vi "Actor Core.vi"(8 "error in":errorcluster, 11 "Nested in":refnum<class "Coins.lvclass">) -> (0 "error out":errorcluster, 3 "Actor out":refnum<class "Actor.lvclass">)   [LabVIEW 2020, in "Coins.lvlib" / "Coins.lvclass"]
doc: "(<B>Filename</B>: Actor Framework.lvlib:Actor.lvclass:Actor Core.vi)\n\nReceives messages to the actor, reacts to them, and initiates any error handling that may shut the actor down.\n\nDescendant classes may override this VI to append parallel tasks for the actor to complete while it handles messages. Overrides use the Call Parent Method node."
uses:
  Coins.lvclass
  C:/Program Files (x86)/National Instruments/LabVIEW 2020/vi.lib/ActorFramework/Actor/Actor.lvclass
  <vilib>/ActorFramework/Actor/Actor.lvclass
  Controls/Currency Enum.ctl
  Coins.lvclass/Coins.ctl
  <vilib>/ActorFramework/Actor/Actor.lvclass/Actor.ctl
  <vilib>/ActorFramework/Message Enqueuer/Message Enqueuer.lvclass/Message Enqueuer.ctl
  Coins Messages/UpdateCoinArray Msg/UpdateCoinArray Msg.lvclass/UpdateCoinArray Msg.ctl
  Coins Messages/AddCredit Msg/AddCredit Msg.lvclass/AddCredit Msg.ctl
  <vilib>/ActorFramework/Message Enqueuer/Init from Existing Queue.vi
  <vilib>/ActorFramework/Message Enqueuer/Enqueue.vi
  <vilib>/ActorFramework/Stop Msg/Stop Msg.lvclass
  C:/Program Files (x86)/National Instruments/LabVIEW 2020/vi.lib/ActorFramework/Message/Message.lvclass
  Coins Messages/UpdateCoinArray Msg/UpdateCoinArray Msg.lvclass
  Coins Messages/AddCredit Msg/AddCredit Msg.lvclass
  Coins Messages/CancelPurchase Msg/CancelPurchase Msg.lvclass
  <vilib>/ActorFramework/Message Priority Queue/Priority Enqueue.vi
  <vilib>/ActorFramework/Message Enqueuer/Message Enqueuer.lvclass
panel:
  in  "Coins Cluster":T1
  out "Currency":T2
  in  "Cancel Button":bool
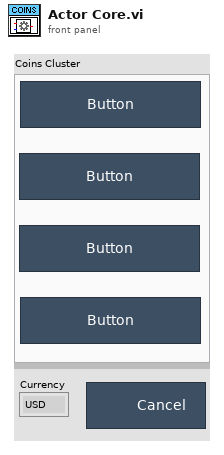
[diagram p1: front panel]
types:
  T1 = cluster{"Coin 1":bool, "Coin 2":bool, "Coin 3":bool, "Coin 4":bool}
  T2 = typedef "Currency Enum.ctl" = enum16{"USD", "MXN", "EUR"}
  T3 = cluster{"Stop":refnum<user-event>, "Currency":refnum<user-event>}
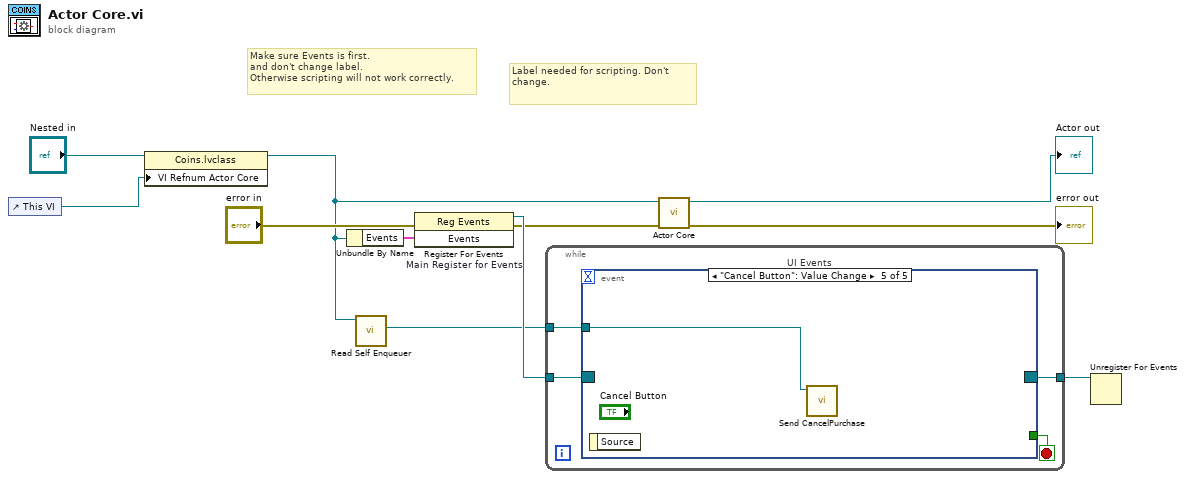
[diagram p0: block diagram]
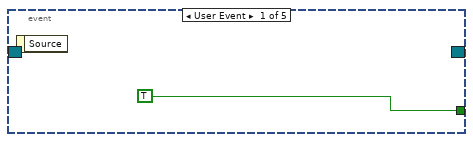
[diagram p2: hidden frame]
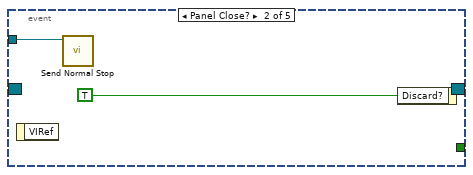
[diagram p3: hidden frame]
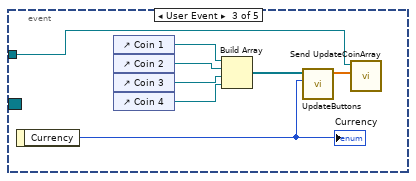
[diagram p4: hidden frame]
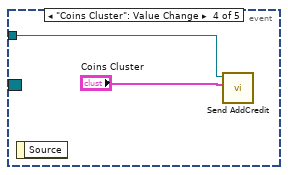
[diagram p5: hidden frame]
diagram:
  # "Label needed for scripting. Don't change."
  # "Make sure Events is first.\nand don't change label.\nOtherwise scripting will not work correctly."
  n1 = control-ref of="This VI"() -> (w1:refnum<vi>)
  n2 = property class="Coins.lvclass"(reference="Nested in", "VI Refnum Actor Core"=w1) -> (reference out=w2:refnum<class "Coins.lvclass">)  [unwired: 1 in, 1 out]
  n3 = Unbundle By Name(w2) -> ("Events"=w8:T3)
  n4 = call <vilib>:"Read Self Enqueuer.vi"("Actor"=w2) -> ("Self Enqueuer"=w5:refnum<class "Message Enqueuer.lvclass">)  [unwired: 10 in]
  n5 = register-events "Main Register for Events"(error in="error in", w8) -> (reference out=w9:refnum<event-registration>, error out=w3:errorcluster)  [unwired: 1 in]
  n6 = while {
    tunnel: w9 -> [w15]
    tunnel: [w13] -> w7
    tunnel: w5 -> [w12]
    stop <- w14 stop-if-true
    n7 = event "UI Events" shown="[4] \"Cancel Button\": Value Change" {
      selector: w15 -> [_ _ _ _ _]
      dyn-events: [_ _ _ _ _] -> w13
      timeout: _ -> [_ _ _ _ _]
      tunnel: [TRUE _ _ _ _] -> w14
      tunnel: w12 -> [_ w17 w20 w28 w29]
      event User Event {
        n8 = event-data() -> ()  [unwired: 1 in, 1 out]
      }
      event Panel Close? {
        n9 = event-data() -> ()  [unwired: 1 in, 1 out]
        n10 = call <vilib>:"Send Normal Stop.vi"("Message Enqueuer"=w17) -> ()  [unwired: 10 in, 1 out]
        n11 = event-data("Discard?"=TRUE) -> ()  [unwired: 1 in, 1 out]
      }
      event User Event {
        n12 = event-data() -> ("Currency"=w21:T2)  [unwired: 1 in]
        "Currency" <- w21
        n13 = control-ref of="Coin 1"() -> (w26:refnum<vi>)
        n14 = control-ref of="Coin 2"() -> (w25:refnum<vi>)
        n15 = control-ref of="Coin 3"() -> (w24:refnum<vi>)
        n16 = control-ref of="Coin 4"() -> (w23:refnum<vi>)
        n17 = Build Array(w26, w25, w24, w23) -> (w22:refnum<vi>[])
        n18 = call "UpdateButtons.vi"("Currency"=w21, "Array"=w22) -> ("Values Array"=w19:dbl[])  [unwired: 9 in]
        n19 = call "Send UpdateCoinArray.vi"("Coins Values"=w19, "Message Enqueuer"=w20) -> ()  [unwired: 8 in, 2 out]
      }
      event "Coins Cluster": Value Change {
        n20 = event-data() -> ()  [unwired: 1 in, 1 out]
        n21 = call "Send AddCredit.vi"("Coins Cluster"="Coins Cluster", "Message Enqueuer"=w28) -> ()  [unwired: 8 in, 2 out]
      }
      event "Cancel Button": Value Change {
        n22 = event-data() -> ()  [unwired: 1 in, 1 out]
        n23 = call "Send CancelPurchase.vi"("Message Enqueuer"=w29) -> ()  [unwired: 9 in, 2 out]
      }
    }
  }
  n24 = call-parent "Actor Core.vi"("error in"=w3, "Actor in"=w2) -> ("error out"=→"error out":errorcluster, "Actor out"=→"Actor out":refnum<class "Actor.lvclass">)  [unwired: 8 in]
  n25 = Unregister For Events(event registration refnum=w7) -> ()  [unwired: 1 in, 1 out]
